vi "001 Funcions diverses arrays.vi"() -> ()   [LabVIEW 2019]
panel:
  out "appended array":i32[](array[numeric])
  in  "elements":i32=3
  in  "índex inici":i32=2
  in  "element":i32=7
  in  "stop":bool
  out "index of element":i32
  out "subarray":i32[](array[numeric])
  out "initialized array":dbl[](array[numeric])
  out "array w/ subset deleted":i32[](array[numeric])
  out "Element":dbl
  out "Tamany":dbl
  # "Et fa un sub-array des de la \nposició que vulguis i fins on \nvulguis"
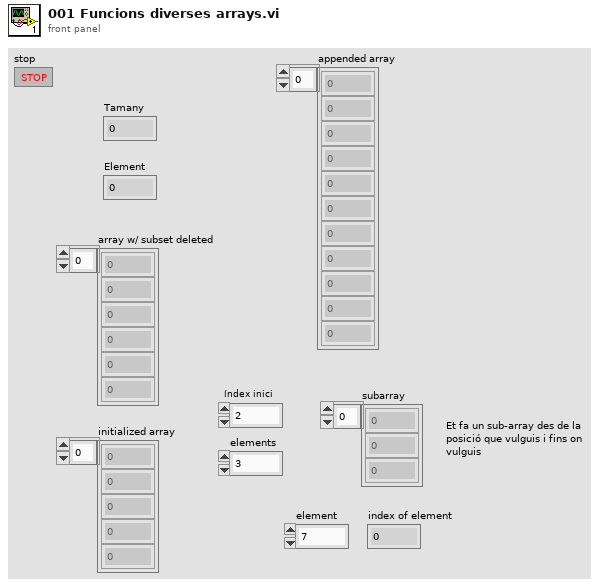
[diagram p1: front panel]
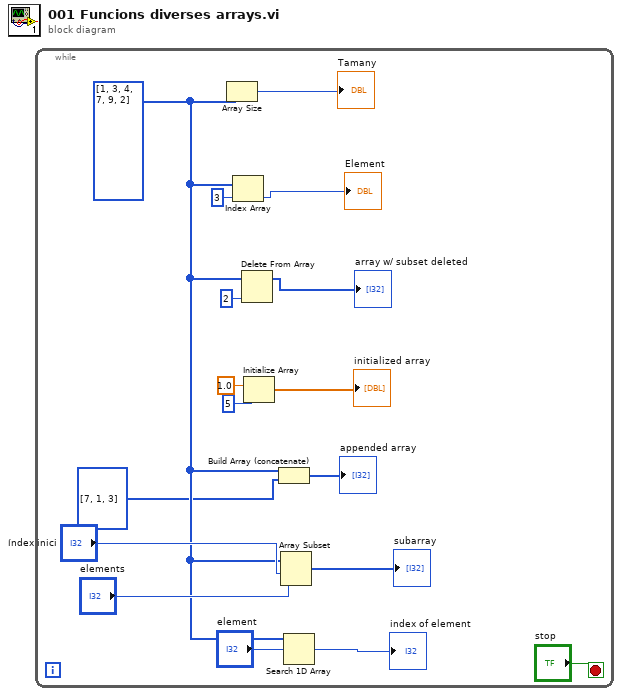
[diagram p0: block diagram]
diagram:
  n1 = while {
    stop <- "stop" stop-if-true
    w6 = i32[] [1, 3, 4, 7, 9, 2] ("Array")
    n2 = Array Size(array=w6) -> (size(s)=→"Tamany":i32)
    n3 = Index Array "Index Array"(array=w6, index=3) -> (element=→"Element":i32)
    n4 = Delete From Array "Delete From Array"(array=w6, index=2) -> (array with subset deleted=→"array w/ subset deleted":i32[])  [unwired: 1 in, 1 out]
    n5 = Initialize Array "Initialize Array"(1.0 ("element"), 5 ("dimension size")) -> (→"initialized array":dbl[])
    n6 = Build Array (concatenate) "Build Array"(w6, i32[] [7, 1, 3] ("element")) -> (→"appended array":i32[])
    n7 = Array Subset "Array Subset"(array=w6, index="índex inici", length="elements") -> (→"subarray":i32[])
    n8 = Search 1D Array(1D array=w6, element="element") -> (index of element=→"index of element":i32)  [unwired: 1 in]
  }
